vi "OM_ToLabVIEW.vi"(8 "error in (no error)":errorcluster, 10 "DbRow":variant, 11 "ObjectLUT in":refnum<class "ObjectLUT.lvclass">) -> (0 "error out":errorcluster, 1 "found":bool, 3 "ObjectLUT out":refnum<class "ObjectLUT.lvclass">)   [LabVIEW 2020, in "ORM_lib.lvlib" / "ObjectLUT.lvclass"]
uses:
  ObjectLUT.lvclass
  ObjectLUT.lvclass/ObjectLUT.ctl
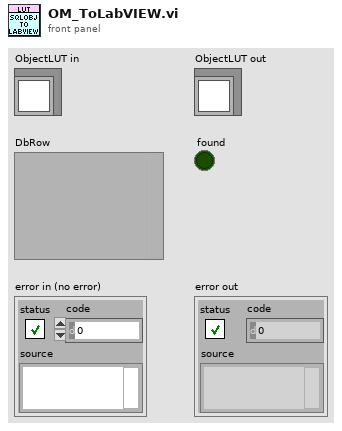
[diagram p1: front panel]
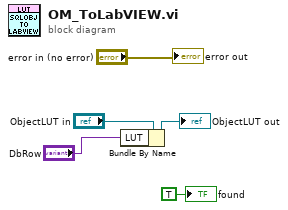
[diagram p0: block diagram]
diagram:
  n1 = Bundle By Name(cluster="ObjectLUT in", "LUT"="DbRow") -> (→"ObjectLUT out":refnum<class "ObjectLUT.lvclass">)
  "error out" <- "error in (no error)"
  "found" <- TRUE ("found")
